vi "Position (Read).vi"(6 "ISOBUS address":T3=-1 caption="ISOBUS address (-1)", 8 "error in":errorcluster, 11 "Mercury Reference In":T4) -> (0 "error out":errorcluster, 1 "Unit":T1, 2 "Position":u32, 3 "Mercury Reference Out":T4, 4 "Valid?":T2)   [LabVIEW 2015, in "Mercury iXX.lvlib" / "Auxiliary.lvlib"]
doc: "Acquire the current position of the stepper motor."
uses:
  Auxiliary.lvlib
  Controls/Mercury Reference.ctl
  Controls/Comms Transport Layer.ctl
  Private/Controls/Query Dynamic Reference.ctl
  Controls/ISOBus Address.ctl
  Controls/Is Valid LED.ctl
  Controls/Unit String.ctl
  Private/Controls/Command Verbs.ctl
  Mercury iXX.lvlib
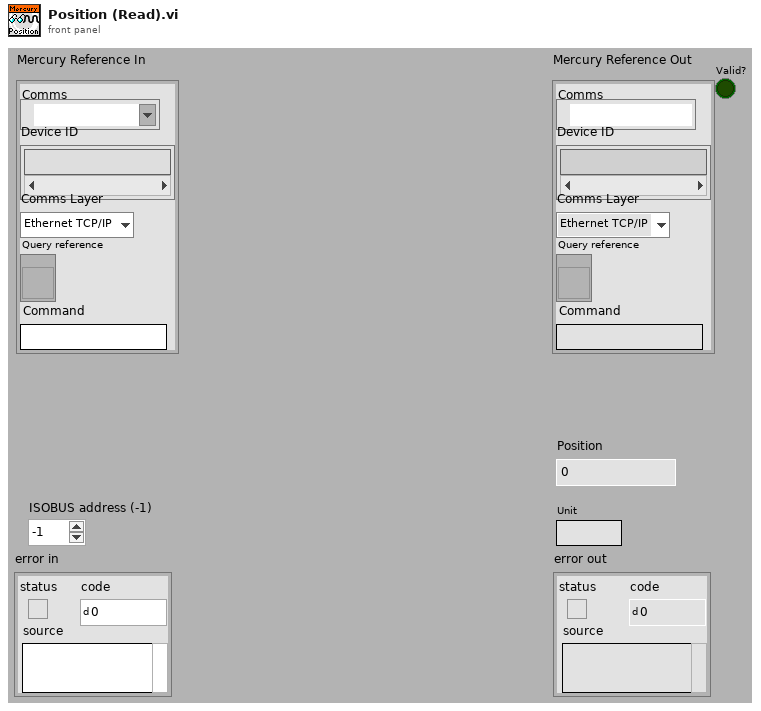
[diagram p1: front panel]
types:
  T1 = typedef "Mercury iXX.lvlib/Unit String.ctl" = string
  T2 = typedef "Mercury iXX.lvlib/Is Valid LED.ctl" = bool
  T3 = typedef "Mercury iXX.lvlib/ISOBus Address.ctl" = i32
  T4 = typedef "Mercury iXX.lvlib/Mercury Reference.ctl" = cluster{"Comms":refnum<visa-resource-name>, "Device ID":string[], "Comms Layer":T5, "Command":string, "Query reference":T6}
  T5 = typedef "Mercury iXX.lvlib/Comms Transport Layer.ctl" = enum16{"Ethernet TCP/IP", "USB", "ISOBus - RS-232", "GPIB"}
  T6 = typedef "Mercury iXX.lvlib/Query Dynamic Reference.ctl" = refnum<vi>
  T7 = typedef "Mercury iXX.lvlib/Command Verbs.ctl" = string
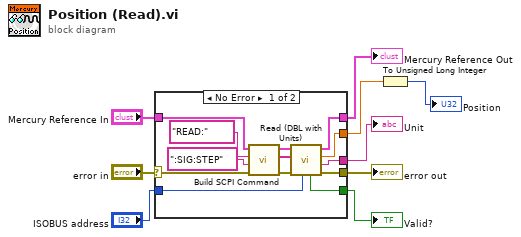
[diagram p0: block diagram]
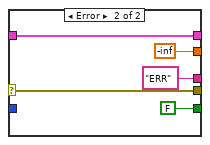
[diagram p2: hidden frame]
diagram:
  n1 = case shown="No Error" "error in" {
    selector: "error in" -> [w15 w26]
    tunnel: "Mercury Reference In" -> [w16 w27]
    tunnel: [w22 w26] -> w3
    tunnel: [w21 w27] -> w6
    tunnel: "ISOBUS address" -> [w20 _]
    tunnel: [w19 T2 FALSE ("Valid?")] -> w5
    tunnel: [w18 -inf] -> w2
    tunnel: [w17 T1 "ERR" ("Unit")] -> w4
    frame No Error {
      n2 = call "Build SCPI Command.vi"("error in"=w15, "Noun(s)"=":SIG:STEP" ("Command"), "Verb"=T7 "READ:", "Mercury Reference In"=w16) -> ("error out"=w11:errorcluster, "SCPI Message(s)"=w10:string[], "Mercury Reference Out"=w14:T4)  [unwired: 5 out]
      n3 = call "Read (DBL with Units).vi"("ISOBUS address"=w20, "error in"=w11, "SCPI Message(s)"=w10, "Mercury Reference In"=w14) -> ("error out"=w22:errorcluster, "Unit"=w17:T1, "Data (Dbl)"=w18:dbl, "Mercury Reference Out"=w21:T4, "Valid?"=w19:T2)  [unwired: 3 out]
    }
    frame Error {
    }
  }
  "Mercury Reference Out" <- w6
  "Valid?" <- w5
  "error out" <- w3
  "Unit" <- w4
  n4 = To Unsigned Long Integer(number=w2) -> (unsigned 32bit integer=→"Position":u32)
